vi "Smooth Arrray.vi"(9 "smooth size":dbl=10.0, 11 "Raw Array":dbl[](array[numeric])) -> (3 "Smoothed Array":dbl[](array[numeric]))   [LabVIEW 2012]
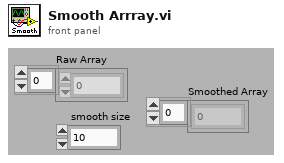
[diagram p1: front panel]
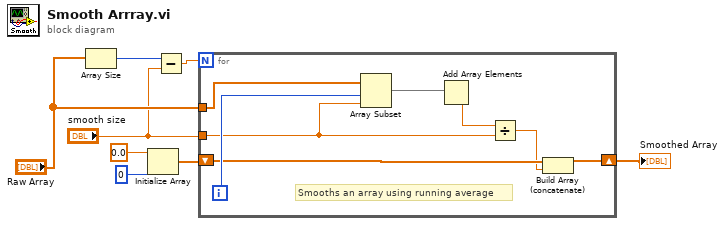
[diagram p0: block diagram]
diagram:
  n1 = Array Size(array="Raw Array") -> (size(s)=w6:i32)
  n2 = Initialize Array(0.0, 0) -> (w2:dbl[])
  n3 = Subtract(x=w6, y="smooth size") -> (x-y=w5:dbl)
  n4 = for {
    N: w5 -> [_]
    tunnel: "Raw Array" -> [w16]
    tunnel: "smooth size" -> [w9]
    shift-right: [w10] -> w1
    shift-left: w2 -> [w12]
    i -> [w15]
    # "Smooths an array using running average"
    n5 = Array Subset(array=w16, index=w15, length=w9) -> (w13:dbl[])
    n6 = Add Array Elements(numeric array=w13) -> (sum=w14:dbl)
    n7 = Divide(x=w14, y=w9) -> (x/y=w11:dbl)
    n8 = Build Array (concatenate)(w12, w11) -> (w10:dbl[])
  }
  "Smoothed Array" <- w1
